vi "Begin.vi"(8 "error in":errorcluster) -> (0 "error out":errorcluster)   [LabVIEW 2016]
doc: "Called before other user functions, this VI is expected to open initial I/O refnums, load in file data, and do all program initialization. Notice that the <B>error out</B> terminal is simply used for data flow. Wiring it to other structures or subVIs ensures that this VI runs first."
uses:
  <vilib>/Rock Robotics/WPI/DriverStation/WPI_DriverStationRobotMode2.ctl
  <vilib>/Rock Robotics/WPI/Joystick/WPI_JoystickDeviceEnum.ctl
  <vilib>/Rock Robotics/SystemInterfaces/DIO/FPGA_DIOPWMChannel.ctl
  <vilib>/Rock Robotics/SystemInterfaces/DIO/FPGA_DIOChannel.ctl
  <vilib>/Rock Robotics/WPI/Solenoid/WPI_SolenoidChannel.ctl
  Robot Global Data.vi
  <vilib>/Rock Robotics/WPI/Solenoid/WPI_SolenoidOpenSingle.vi
  <vilib>/Rock Robotics/WPI/Counter/WPI_CounterDigitalInputToDigitalSource.vi
  <vilib>/Rock Robotics/WPI/Counter/WPI_CounterOpen UpDown Mode.vi
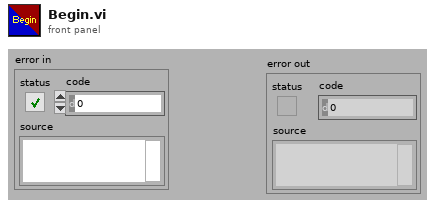
[diagram p1: front panel]
types:
  T1 = enum16{"Rising Edge", "Falling Edge", "Raising & Falling Edge", "Disabled"}
  T2 = typedef "FPGA_DIOChannel.ctl" = enum8{"DIO 0", "DIO 1", "DIO 2", "DIO 3", "DIO 4", "DIO 5", "DIO 6", "DIO 7", "DIO 8", "DIO 9", "DIO MXP 0", "DIO MXP 1", "DIO MXP 2", "DIO MXP 3", "DIO MXP 4", "DIO MXP 5", "DIO MXP 6", "DIO MXP 7", "DIO MXP 8", "DIO MXP 9", "DIO MXP 10", "DIO MXP 11", "DIO MXP 12", "DIO MXP 13", "DIO MXP 14", "DIO MXP 15", "SPI Port CS1", "SPI Port CS2", "SPI Port CS3", "SPI Port MISO", "SPI Port MOSI", "Invalid"}
  T3 = typedef "WPI_SolenoidChannel.ctl" = enum8{"Solenoid 0", "Solenoid 1", "Solenoid 2", "Solenoid 3", "Solenoid 4", "Solenoid 5", "Solenoid 6", "Solenoid 7", "Invalid"}
  T4 = typedef "FPGA_DIOPWMChannel.ctl" = enum8{"PWM 0", "PWM 1", "PWM 2", "PWM 3", "PWM 4", "PWM 5", "PWM 6", "PWM 7", "PWM 8", "PWM 9", "PWM MXP 0", "PWM MXP 1", "PWM MXP 2", "PWM MXP 3", "PWM MXP 4", "PWM MXP 5", "PWM MXP 6", "PWM MXP 7", "PWM MXP 8", "PWM MXP 9", "Invalid"}
  T5 = typedef "WPI_JoystickDeviceEnum.ctl" = enum16{"USB 0", "USB 1", "USB 2", "USB 3", "USB 4", "USB 5"}
  T6 = typedef "WPI_DriverStationRobotMode2.ctl" = enum16{"Autonomous Disabled", "Autonomous Enabled", "Teleop Disabled", "Teleop Enabled", "Disconnected", "Finish", "Test Disabled", "Test Enabled", "Emergency Stopped"}
  T7 = typedef "WPI_JoystickDevRef.ctl" = cluster{"Device":T5}
  T8 = typedef "WPI_DigitalInputDevRef.ctl" = cluster{"DevStatus":errorcluster, "DIO Channel":T2}
  T9 = typedef "FPGA_CounterEncoderSourceConvertionLVSourceType.ctl" = cluster{"DevStatus":errorcluster, "AnalogTriggerMode?":bool, "DigitalMode":cluster{"DIO Channel":T10}, "AnalogTriggerMode":cluster{"AnalogTriggerIndex":T11, "OutputType":T12}}
  T10 = typedef "FPGA_DIODigitalSourceChannel.ctl" = enum8{"DIO 0", "DIO 1", "DIO 2", "DIO 3", "DIO 4", "DIO 5", "DIO 6", "DIO 7", "DIO 8", "DIO 9", "DIO MXP 0", "DIO MXP 1", "DIO MXP 2", "DIO MXP 3", "DIO MXP 4", "DIO MXP 5", "DIO MXP 6", "DIO MXP 7", "DIO MXP 8", "DIO MXP 9", "DIO MXP 10", "DIO MXP 11", "DIO MXP 12", "DIO MXP 13", "DIO MXP 14", "DIO MXP 15", "Disabled"}
  T11 = typedef "FPGA_AnalogTriggerIndex.ctl" = enum8{"Trig 0", "Trig 1", "Trig 2", "Trig 3", "Trig 4", "Trig 5", "Trig 6", "Trig 7", "Invalid"}
  T12 = typedef "FPGA_AnalogTriggerOutType.ctl" = enum16{"InWindow", "TriggerState", "Rising", "Falling"}
  T13 = typedef "WPI_CounterDevRef.ctl" = cluster{"DevStatus":errorcluster, "CntIndex":T14}
  T14 = typedef "FPGA_CounterCtrSystemIndex.ctl" = enum8{"Ctr 0", "Ctr 1", "Ctr 2", "Ctr 3", "Ctr 4", "Ctr 5", "Ctr 6", "Ctr 7", "Invalid"}
  T15 = typedef "WPI_SolenoidDevRef.ctl" = cluster{"DevStatus":errorcluster, "Pneumatics Control Module":u8, "Forward Solenoid Channel":T3, "Reverse Solenoid Channel":T3}
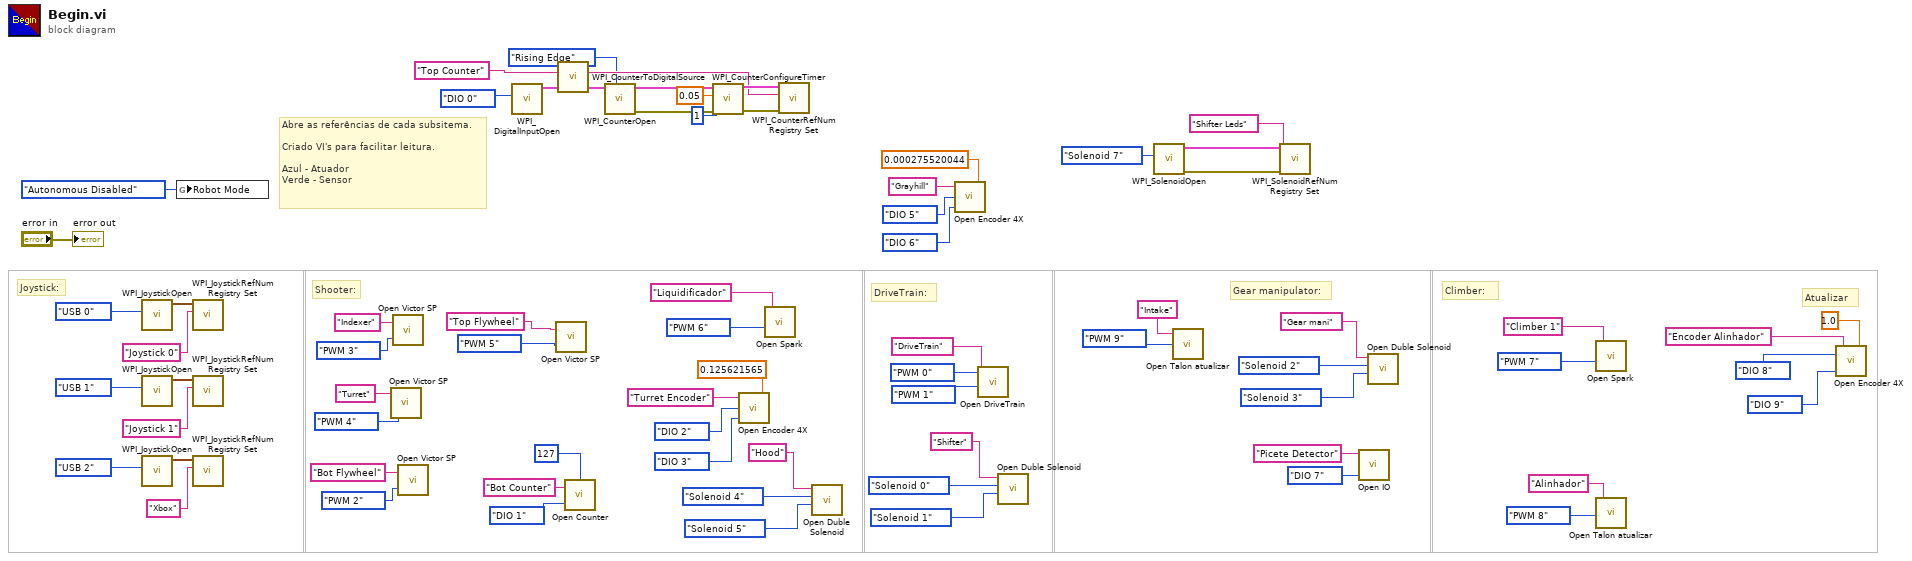
[diagram p0: block diagram]
diagram:
  # "Atualizar"
  # "Climber:"
  # "Gear manipulator:"
  # "DriveTrain:"
  # "Joystick:"
  # "Shooter:"
  # "Abre as referências de cada subsitema.\n\nCriado VI's para facilitar leitura.\n\nAzul - Atuador\nVerde - Sensor"
  n1 = call <vilib>:"WPI_JoystickOpen.vi"("JoystickDevice"=WPI_JoystickDeviceEnum."USB 0") -> ("JoystickDevRef"=w70:T7)  [unwired: 10 in]
  n2 = call <vilib>:"WPI_JoystickOpen.vi"("JoystickDevice"=WPI_JoystickDeviceEnum."USB 1") -> ("JoystickDevRef"=w64:T7)  [unwired: 10 in]
  n3 = call <vilib>:"WPI_JoystickOpen.vi"("JoystickDevice"=WPI_JoystickDeviceEnum."USB 2") -> ("JoystickDevRef"=w63:T7)  [unwired: 10 in]
  n4 = global write "Robot Global Data.vi" "Robot Mode"(WPI_DriverStationRobotMode2."Autonomous Disabled" ("Robot Mode")) -> ()
  n5 = call <vilib>:"WPI_JoystickRefNum Registry Set.vi"("refnum name"="Joystick 0", "JoystickDevRef"=w70) -> ()  [unwired: 8 in, 2 out]
  n6 = call <vilib>:"WPI_JoystickRefNum Registry Set.vi"("refnum name"="Joystick 1", "JoystickDevRef"=w64) -> ()  [unwired: 8 in, 2 out]
  n7 = call <vilib>:"WPI_JoystickRefNum Registry Set.vi"("refnum name"="Xbox", "JoystickDevRef"=w63) -> ()  [unwired: 8 in, 2 out]
  n8 = call "Open Victor SP.vi"("PWM Channel"=FPGA_DIOPWMChannel."PWM 4", "refnum name"="Turret") -> ()  [unwired: 1 in]
  n9 = call "Open Victor SP.vi"("PWM Channel"=FPGA_DIOPWMChannel."PWM 3", "refnum name"="Indexer") -> ()  [unwired: 1 in]
  n10 = call "Open Victor SP.vi"("PWM Channel"=FPGA_DIOPWMChannel."PWM 2", "refnum name"="Bot Flywheel") -> ()  [unwired: 1 in]
  n11 = call <vilib>:"WPI_DigitalInputOpen.vi"("DIO Channel"=FPGA_DIOChannel."DIO 0" ("Source")) -> ("DigitalInputDevRef"=w7:T8)  [unwired: 1 in, 9 out]
  n12 = call "Open Victor SP.vi"("PWM Channel"=FPGA_DIOPWMChannel."PWM 5", "refnum name"="Top Flywheel") -> ()  [unwired: 1 in]
  n13 = call-poly <vilib>:"WPI_CounterToDigitalSource.vi"("DigitalInputDevRef"=w7) -> ("Digital Source"=w6:T9)  [unwired: 6 out]
  n14 = call "Open Counter.vi"("Number Samples to Average"=u8 127, "Source"=FPGA_DIOChannel."DIO 1", "refnum name"="Bot Counter") -> ()  [unwired: 1 in]
  n15 = call-poly <vilib>:"WPI_CounterOpen.vi"("UpEdge"=T1."Rising Edge", "Up Source"=w6) -> ("error out"=w9:errorcluster, "CounterDevRef"=w8:T13)  [unwired: 5 in, 3 out]
  n16 = call <vilib>:"WPI_CounterConfigureTimer.vi"("error in (no error)"=w9, "Number Samples to Average"=u8 1, "MaxPeriod (sec)"=0.05, "CounterDevRef in"=w8) -> ("error out"=w11:errorcluster, "CounterDevRef out"=w10:T13)  [unwired: 6 in]
  n17 = call "Open Encoder 4X.vi"("DistancePerCount"=0.125621565, "B Channel"=FPGA_DIOChannel."DIO 3", "A Channel"=FPGA_DIOChannel."DIO 2", "refnum name"="Turret Encoder") -> ()  [unwired: 1 in]
  n18 = call "Open Spark.vi"("PWM Channel"=FPGA_DIOPWMChannel."PWM 6", "refnum name"="Liquidificador") -> ()  [unwired: 1 in]
  n19 = call <vilib>:"WPI_CounterRefNum Registry Set.vi"("error in (no error)"=w11, "refnum name"="Top Counter", "CounterDevRef"=w10) -> ()  [unwired: 7 in, 2 out]
  n20 = call "Open Duble Solenoid.vi"("Reverse Solenoid Channel"=WPI_SolenoidChannel."Solenoid 5", "Forward Solenoid Channel"=WPI_SolenoidChannel."Solenoid 4", "refnum name"="Hood") -> ()  [unwired: 9 in]
  n21 = call "Open Encoder 4X.vi"("DistancePerCount"=0.000275520044, "B Channel"=FPGA_DIOChannel."DIO 6", "A Channel"=FPGA_DIOChannel."DIO 5", "refnum name"="Grayhill") -> ()  [unwired: 1 in]
  n22 = call "Open DriveTrain.vi"("PWM Channel 2"=FPGA_DIOPWMChannel."PWM 1", "PWM Channel"=FPGA_DIOPWMChannel."PWM 0", "refnum name"="DriveTrain") -> ()  [unwired: 9 in]
  n23 = call "Open Duble Solenoid.vi"("Reverse Solenoid Channel"=WPI_SolenoidChannel."Solenoid 1", "Forward Solenoid Channel"=WPI_SolenoidChannel."Solenoid 0", "refnum name"="Shifter") -> ()  [unwired: 9 in]
  n24 = call-poly <vilib>:"WPI_SolenoidOpen.vi"("Solenoid Channel"=WPI_SolenoidChannel."Solenoid 7") -> ("error out"=w14:errorcluster, "SolenoidDevRef"=w15:T15)  [unwired: 9 in]
  n25 = call "Open Talon atualizar.vi"("PWM Channel"=FPGA_DIOPWMChannel."PWM 9", "refnum name"="Intake") -> ()  [unwired: 7 in]
  n26 = call <vilib>:"WPI_SolenoidRefNum Registry Set.vi"("error in (no error)"=w14, "refnum name"="Shifter Leds", "SolenoidDevRef"=w15) -> ()  [unwired: 7 in, 2 out]
  n27 = call "Open IO.vi"("DIO Channel"=FPGA_DIOChannel."DIO 7", "refnum name"="Picete Detector") -> ()  [unwired: 10 in]
  n28 = call "Open Duble Solenoid.vi"("Reverse Solenoid Channel"=WPI_SolenoidChannel."Solenoid 3", "Forward Solenoid Channel"=WPI_SolenoidChannel."Solenoid 2", "refnum name"="Gear mani") -> ()  [unwired: 9 in]
  n29 = call "Open Spark.vi"("PWM Channel"=FPGA_DIOPWMChannel."PWM 7", "refnum name"="Climber 1") -> ()  [unwired: 1 in]
  n30 = call "Open Talon atualizar.vi"("PWM Channel"=FPGA_DIOPWMChannel."PWM 8", "refnum name"="Alinhador") -> ()  [unwired: 7 in]
  n31 = call "Open Encoder 4X.vi"("DistancePerCount"=1.0, "B Channel"=FPGA_DIOChannel."DIO 9", "A Channel"=FPGA_DIOChannel."DIO 8", "refnum name"="Encoder Alinhador") -> ()  [unwired: 1 in]
  "error out" <- "error in"
